vi "No GyroScope Acc Test.vi"() -> ()   [LabVIEW 2019]
uses:
  <vilib>/Platform/TimedLoop/XDataNode/timing_clust.ctl
  <vilib>/Platform/TimedLoop/XDataNode/nitl_modes.ctl
  <vilib>/Platform/TimedLoop/XDataNode/wakeup.ctl
  <vilib>/FPGAPlugInAG/cRIO-9065/niLvFpga_Open_cRIO-9065.vi
  <vilib>/rvi/interface/common/dynamic/niFpgaDynamicAddResources.vi
  <vilib>/Utility/error.llb/Error Cluster From Error Code.vi
  <vilib>/rvi/errors/niLvFpgaAdjustHostInterfaceError.vi
  <vilib>/FPGAPlugInAG/Dynamic/niLvFpga_Run_Dynamic.vi
  <vilib>/FPGAPlugInAG/Dynamic/niLvFpga_Abort_Dynamic.vi
  <vilib>/platform/TimedLoop/XDataNode/XDataNode.xnode
  <vilib>/rvi/interface/nirviOpenFPGA/nirviOpenFPGA.xnode
  FPGA Bitfiles/crio9065control_FPGATarget_3motionboardtest_jcOy0Y5QmHo.lvbitx
  <vilib>/rvi/interface/nirviReadWriteControl/nirviReadWriteControl.xnode
  <vilib>/rvi/interface/nirviMethod/nirviMethod.xnode
  NiFpgaLv.dll
  <vilib>/rvi/interface/Simulation/niFpgaSimulationCallBeginRW.vi
  <vilib>/Platform/TimedLoop/XDataNode/XDNodeRunTimeDep.lvlib
  <vilib>/Analysis/NI_AALPro.lvlib
panel:
  out "Axis 3 Real Acceleration Graph":cluster{i32[], "Ideal Acc":dbl[]}[](graph)
  out "Axis 2 Real Acceleration Graph":cluster{i32[], "Ideal Acc":dbl[]}[](graph)
  out "Axis 3 Real Velocity Graph":cluster{i32[], "Ideal Velocity":dbl[]}[](graph)
  out "Axis 2 Real Velocity Graph":cluster{i32[], "Ideal Velocity":dbl[]}[](graph)
  out "Axis 1 Real Acceleration Graph":cluster{i32[], "dX/dt":dbl[]}[](graph)
  out "Axis 1 Real Velocity Graph":cluster{i32[], "Ideal Velocity":dbl[]}[](graph)
  out "Axis 1":cluster{i32[], "Ideal Move":dbl[]}[](graph)
  out "Axis 3":cluster{i32[], "Ideal Move":dbl[]}[](graph)
  out "Axis 2":cluster{i32[], "Ideal Move":dbl[]}[](graph)
  in  "Period":i64=10
  in  "stop":bool
  out "time loop error":errorcluster
  out "Axis 1 速率 (1mm/s)":dbl
  out "Real Period":u32
  out "沖壓":bool
  out "結束了":bool
  out "Voltage\nOutput":dbl
  out "Voltage\nOutput 2":dbl
  out "Voltage\nOutput 3":dbl
  out "Axis 2 速率 (1mm/s)":dbl
  out "Axis 3 速率 (1mm/s)":dbl
  out "shutdown error":errorcluster
  in  "Tab Control":enum32{"Axis Control"}(tab)
  in  "Axis 1~3 Servo on?":bool
  out "Axis 3 Backward Limit":bool
  out "Axis 3 Backward Limit 2":bool
  out "Axis 2 Backward Limit":bool
  out "Axis 2 Backward Limit 2":bool
  in  "Axis 3 Alarm Reset":bool
  in  "Axis 2 Alarm Reset":bool
  in  "Axis 3 Position Reset":bool
  in  "Axis 2 Position Reset":bool
  in  "Axis 1 Alarm Reset":bool
  in  "Axis 1 Position Reset":bool
  in  "Axis 3 Speed":fxp<+/-,64,32>
  in  "Axis 2 Speed":fxp<+/-,64,32>
  out "Axis 3 Encoder Position (Counts)":i32
  out "Axis 2 Encoder Position (Counts)":i32
  out "Axis 1 Encoder Position (Counts)":i32
  in  "Axis 1 Spped":fxp<+/-,64,32>
  in  "Axis 2 Servo on?":bool
  in  "Axis 3 Servo on?":bool
  in  "Axis 1 Servo on?":bool
  out "Axis 1 Forward Limit":bool
  out "Axis 1 Backward Limit":bool
  out "Timed Out?":bool
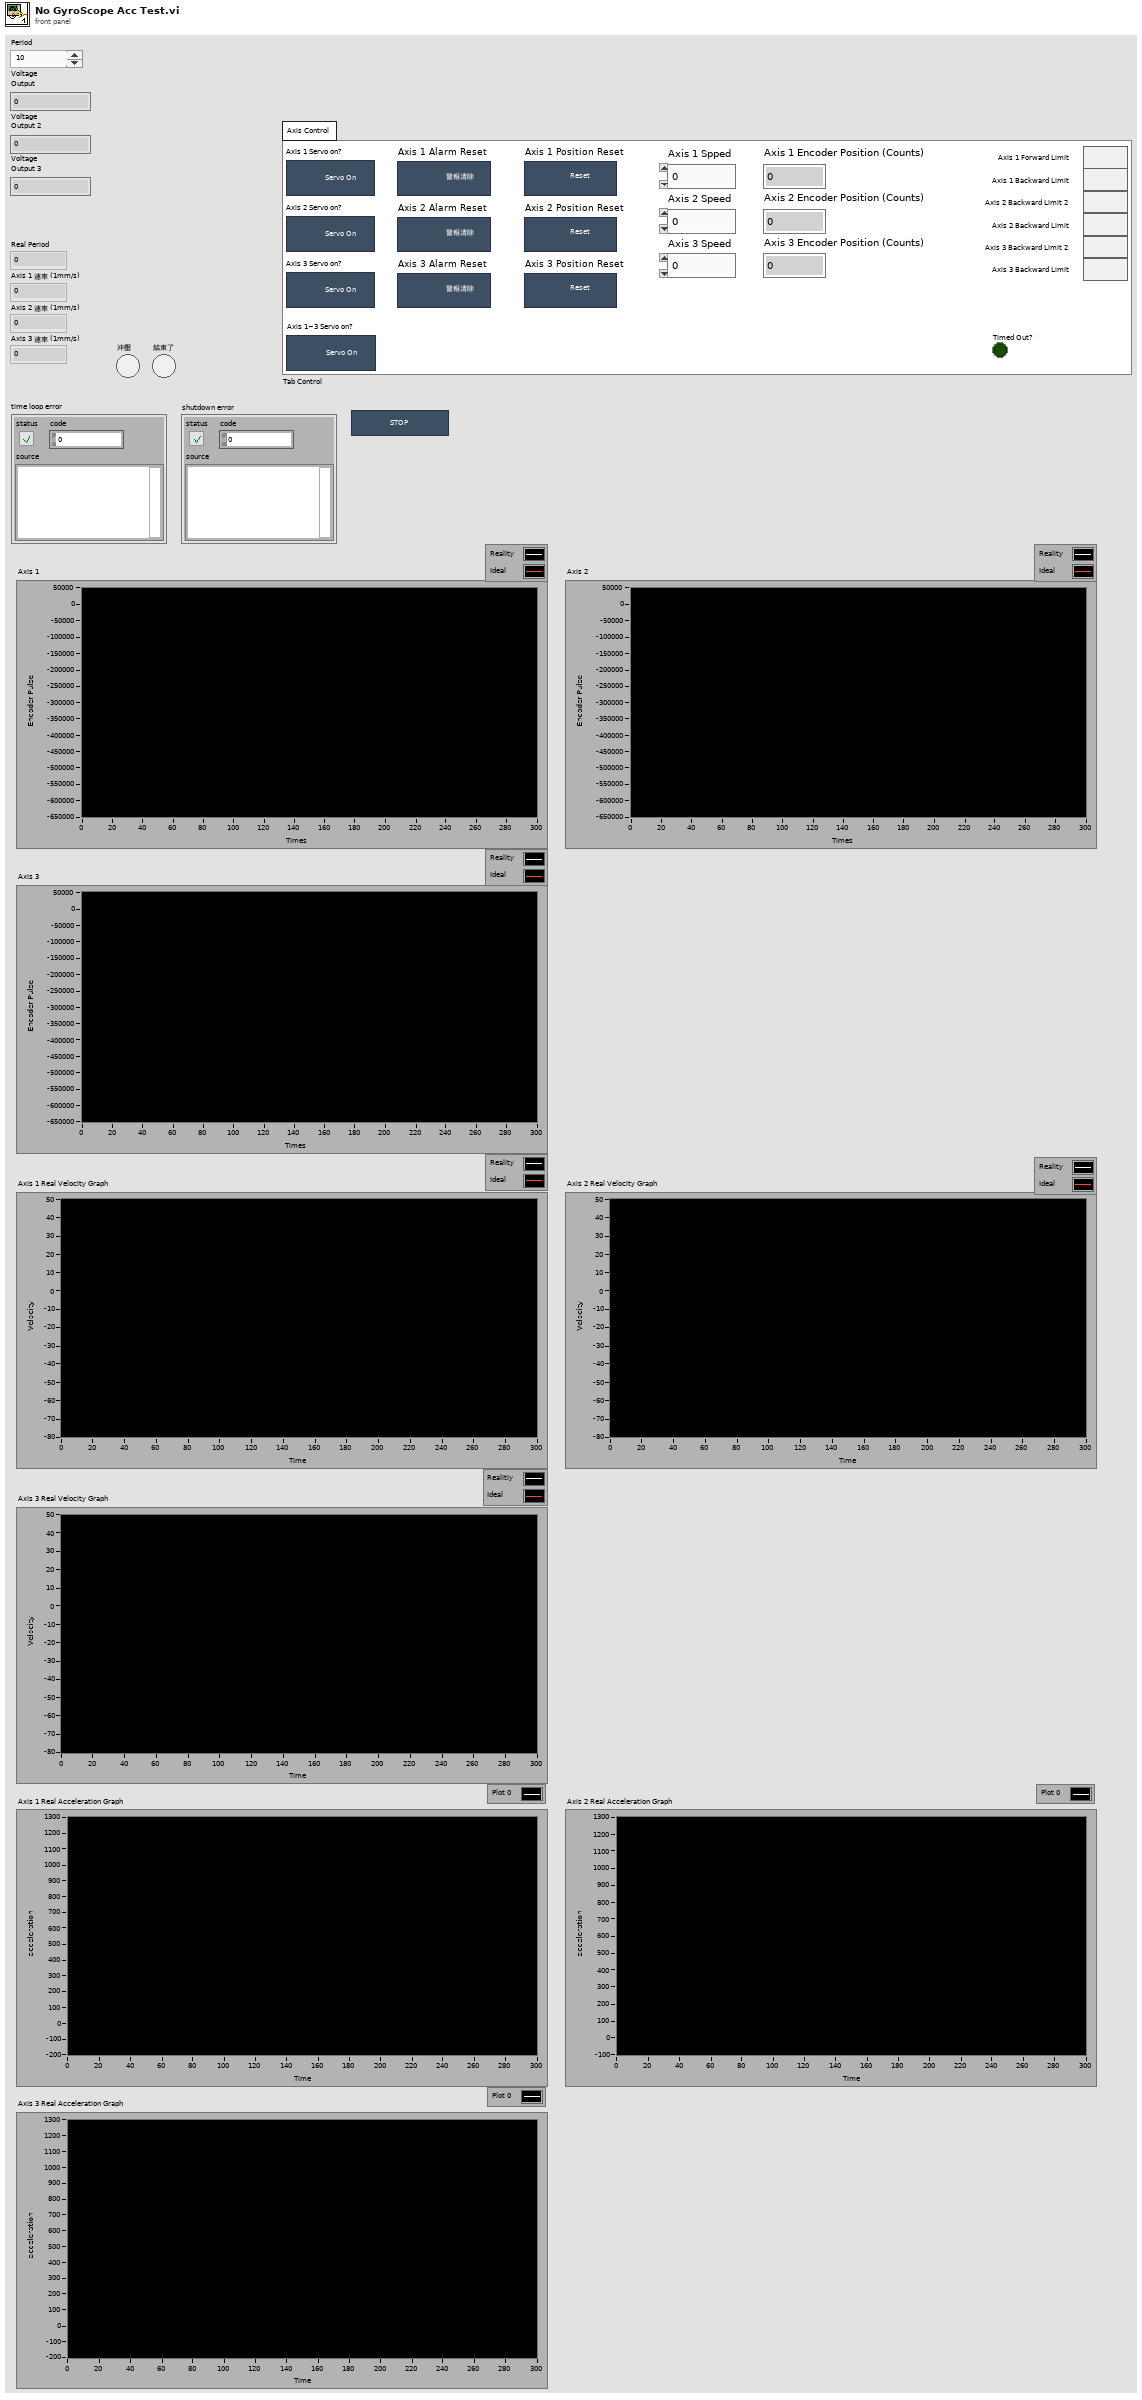
[diagram p1: front panel]
types:
  T1 = enum16{"open", "replace", "create", "open or create", "replace or create", "replace or create with confirmation"}
  T2 = cluster{"Acceleration 1":dbl, "Acceleration 2":dbl, "Acceleration 3":dbl, "Acceleration 4":dbl, "Acceleration 5":dbl, "Acceleration 6":dbl, "Acceleration 7":dbl, "Acceleration 8":dbl}
  T3 = cluster{"Time 1":dbl, "Time 2":dbl, "Time 3":dbl, "Time 4":dbl, "Time 5":dbl, "Time 6":dbl, "Time 7":dbl, "Time 8":dbl}
  T4 = typedef "XDNodeRunTimeDep.lvlib/timing_clust.ctl" = cluster{"Expected End [f-1]":u64, "Actual End [f-1]":u64, "Finished Late? [f-1]":bool, "Expected End [i-1]":u64, "Actual End [i-1]":u64, "Finished Late? [i-1]":bool, "Expected Start [i]":u64, "Actual Start [i]":u64, "Expected Start [f]":u64, "Actual Start [f]":u64, "Source Name":string, "Structure Name":string, "Period":i64, "Deadline":i64, "Offset":i64, "Start":i64, "Priority":i32, "Timeout":i32, "Mode":T5, "Wakeup Reason":T6, "Error":errorcluster, "Source Type":string, "Secondary Source Type":string, "Global End Time":u64, "Global Start Time":u64, "Frame Duration":u64, "Iteration Duration":u64, "Assigned CPU":i32, "I/O Scan Engine Mode":u32}
  T5 = typedef "XDNodeRunTimeDep.lvlib/nitl_modes.ctl" = enum32{"No Change", "Process missed periods, maintain original phase", "Discard missed periods, maintain original phase", "Process missed periods, ignore original phase", "Discard missed periods, ignore original phase"}
  T6 = typedef "XDNodeRunTimeDep.lvlib/wakeup.ctl" = enum32{"Normal", "Aborted", "Asynchronous wakeup", "Timing source error", "Timed loop error", "Timeout"}
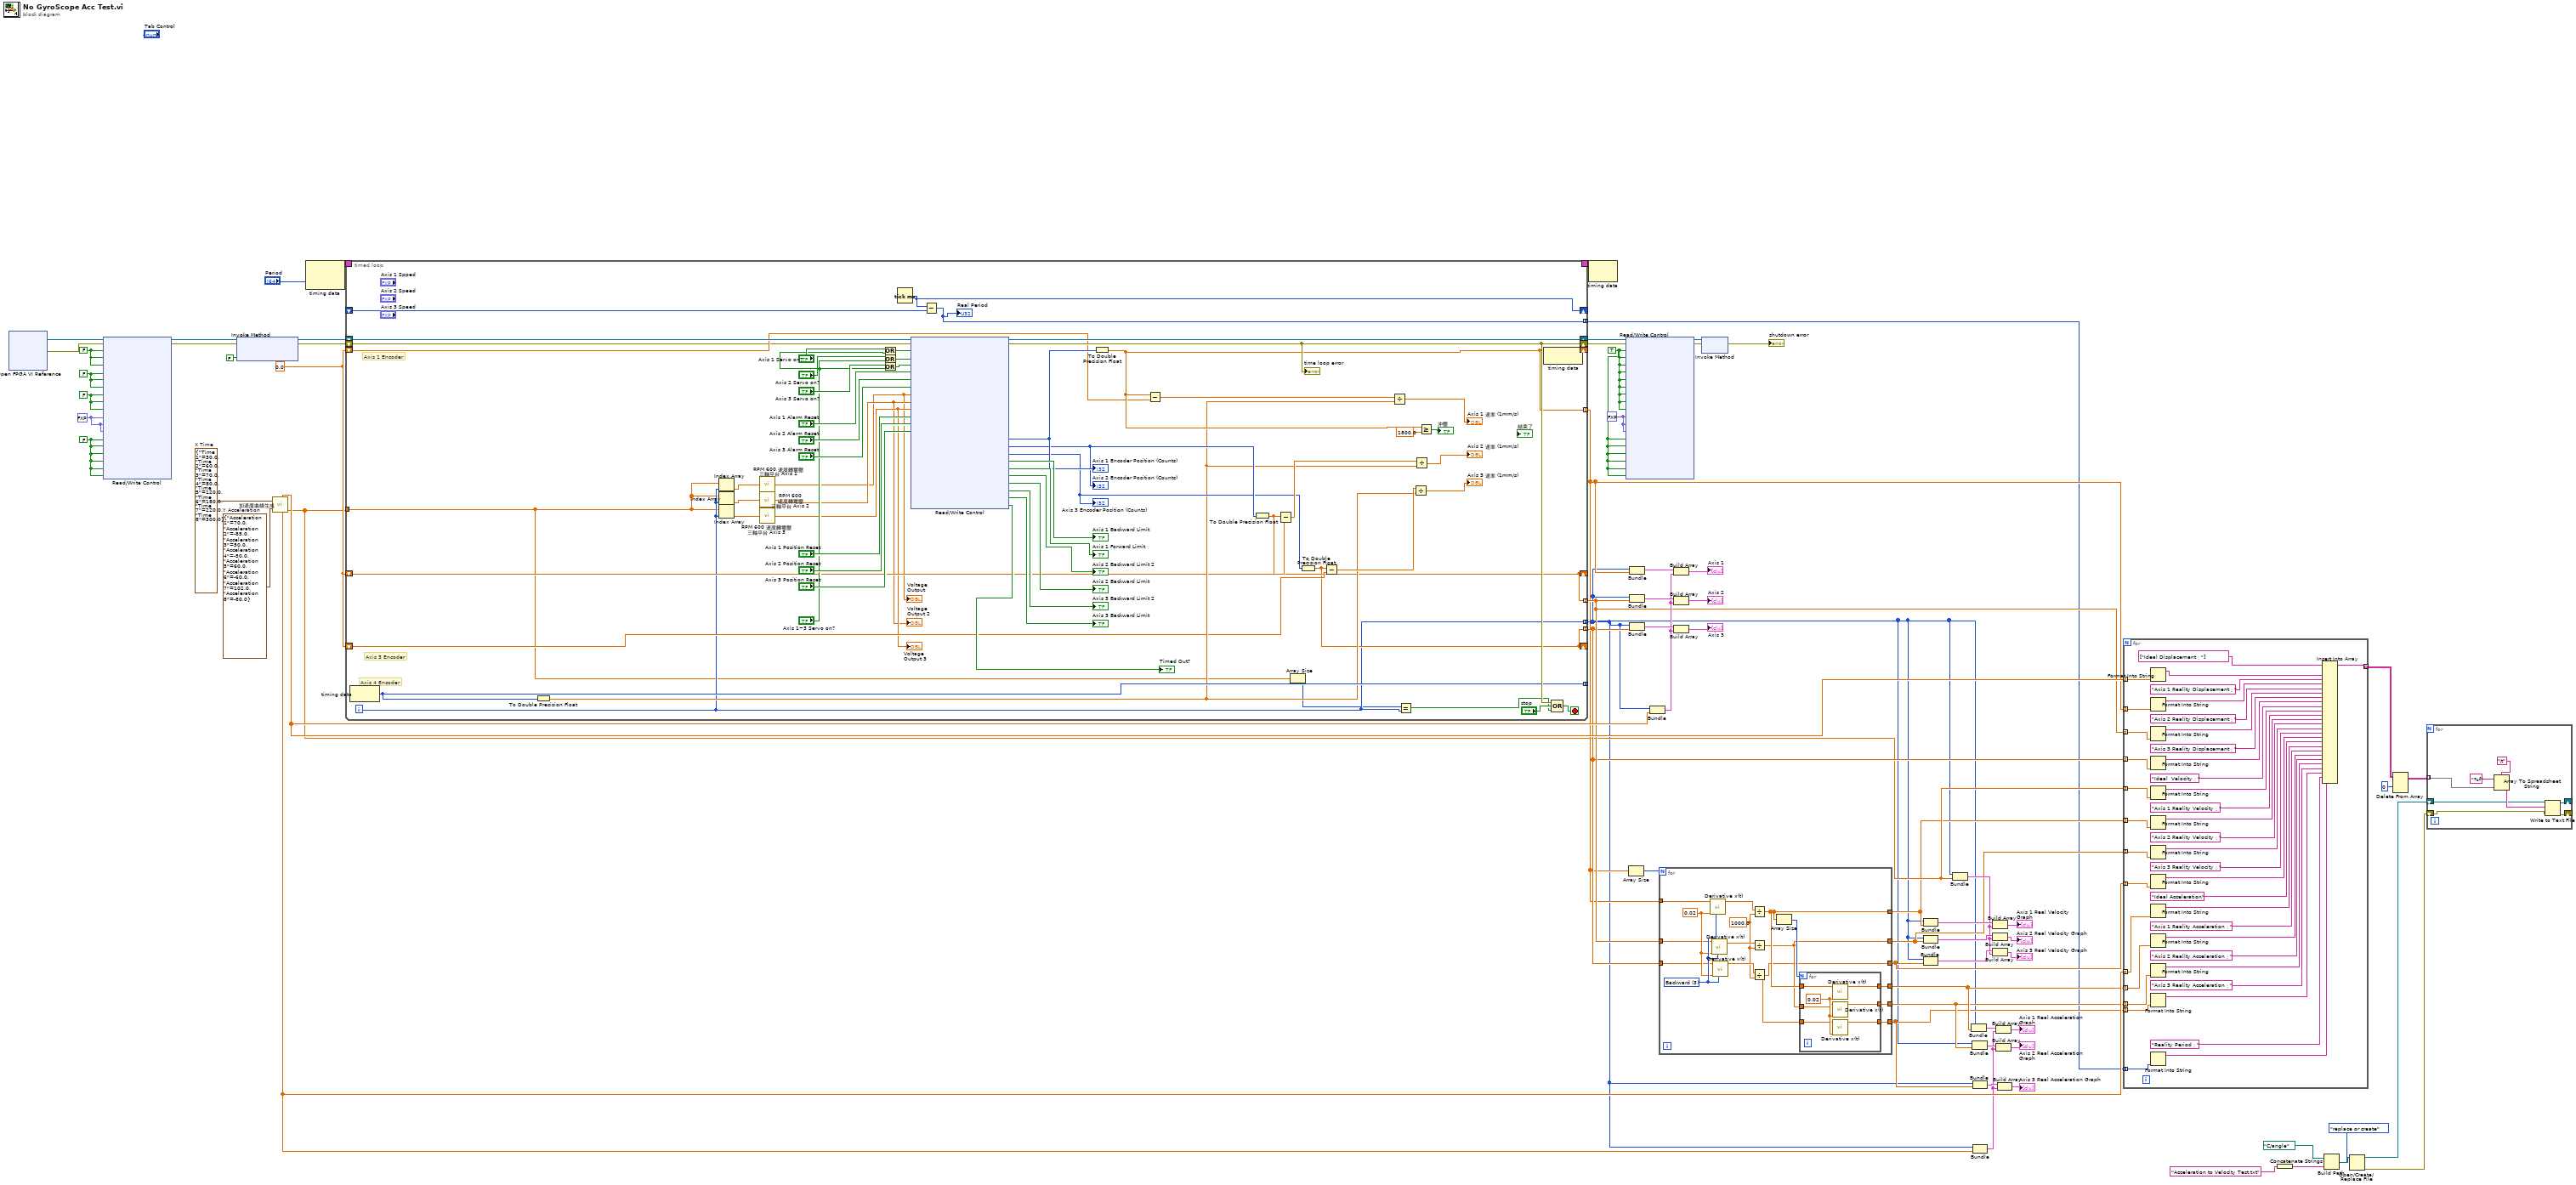
[diagram p0: block diagram]
diagram:
  w48 = T2 {"Acceleration 1"=70.0, "Acceleration 2"=-85.0, "Acceleration 3"=50.0, "Acceleration 4"=-50.0, "Acceleration 5"=60.0, "Acceleration 6"=-60.0, "Acceleration 7"=102.0, "Acceleration 8"=-80.0}  # Y Acceleration
  w50 = T3 {"Time 1"=30.0, "Time 2"=60.0, "Time 3"=70.0, "Time 4"=80.0, "Time 5"=120.0, "Time 6"=180.0, "Time 7"=220.0, "Time 8"=300.0}  # X Time
  w52 = FALSE
  w54 = FALSE
  w60 = 0.0
  w58 = fxp<+,1,1> 0.0
  w57 = TRUE
  w55 = FALSE
  w53 = fxp<+,1,1> 0.0
  w56 = FALSE
  n1 = xnode "Open FPGA VI Reference"() -> ("FPGA VI Reference Out"=w51:refnum<k20>, "error out"=w1:errorcluster)  [unwired: 2 in]
  n2 = xnode "Read/Write Control"("FPGA VI Reference In"=w51, "error in"=w1, "Axis 1 Servo on?"=w56, "Axis 2 Servo on?"=w56, "Axis 3 Servo on?"=w56, "Axis 1 Alarm Reset"=w55, "Axis 2 Alarm Reset"=w55, "Axis 3 Alarm Reset"=w55, "Axis 1 Position Reset"=w54, "Axis 2 Position Reset"=w54, "Axis 3 Position Reset"=w54, "Axis 1 Voltage In"=w53, "Axis 2 Voltage In"=w53, "Axis 3 Voltage In"=w53, "Axis 1 Backward Limit"=w52, "Axis 1 Forward Limit"=w52, "Axis 2 Forward Limit"=w52, "Axis 2 Backward Limit"=w52, "Axis 3 ForWard Limit"=w52, "Axis 3 Backward Limit"=w52) -> ("FPGA VI Reference Out"=w69:refnum<k20>, "error out"=w68:errorcluster)
  n3 = xnode "Invoke Method"("FPGA VI Reference In"=w69, "error in"=w68, "Wait Until Done (F)"=FALSE) -> ("FPGA VI Reference Out"=w66:refnum<k20>, "error out"=w2:errorcluster)
  n4 = call "加速度曲線生成.vi"("X Time"=w50, "Y Velocity"=w48) -> ("Ideal Move"=w26:dbl[], "Ideal Acc"=w9:dbl[], "Ideal Velocity"=w22:dbl[])  [unwired: 3 out]
  n5 = node-c288("Period") -> (w71:T4)  [unwired: 1 in]
  n6 = timed-loop {
    shift-right: [w128] -> w62
    shift-left: w66 -> [w127]
    shift-right: [w95] -> w63
    shift-left: w2 -> [w72]
    timing: w71 -> [_]
    timing-out: [_] -> w70
    shift-right: [w90] -> _
    shift-left: w60 -> [w89]
    tunnel: [w94] -> _ mode=indexing
    shift-right: [w124] -> _
    shift-left: _ -> [w125]
    tunnel: [w84] -> w5 mode=indexing
    shift-right: [w83] -> _
    shift-left: w60 -> [w86]
    shift-right: [w82] -> _
    shift-left: w60 -> [w87]
    tunnel: [w81] -> w3 mode=indexing
    tunnel: [w90] -> w23 mode=indexing
    tunnel: [w83] -> w25 mode=indexing
    tunnel: [w82] -> w24 mode=indexing
    tunnel: w22 -> [w73]
    i -> [w81]
    stop <- w126 stop-if-true
    # "Axis 3 Encoder"
    # "Axis 4 Encoder"
    # "Axis 1 Encoder"
    n7 = node-c288() -> (w94:i64)  [unwired: 1 in]
    n8 = To Double Precision Float(number=w94) -> (double precision float=w88:dbl)
    n9 = Index Array(array=w73, index=w81) -> (element=w78:dbl)
    n10 = Index Array(array=w73, index=w81) -> (element=w77:dbl)
    n11 = Index Array(array=w73, index=w81) -> (element=w79:dbl)
    n12 = call "RPM 600 速度轉電壓 三軸平台 Axis 1.vi"("Speed (1mm/s)"=w78) -> ("Voltage\nOutput"=w74:dbl)
    "Voltage\nOutput" <- w74
    n13 = call "RPM 600 速度轉電壓 三軸平台 Axis 2.vi"("Speed (1mm/s)"=w77) -> ("Voltage\nOutput"=w75:dbl)
    "Voltage\nOutput 2" <- w75
    n14 = call "RPM 600 速度轉電壓 三軸平台 Axis 3.vi"("Speed (1mm/s)"=w79) -> ("Voltage\nOutput"=w76:dbl)
    "Voltage\nOutput 3" <- w76
    n15 = Or(x="Axis 1 Servo on?", y="Axis 1~3 Servo on?") -> (x .or. y?=w107:bool)
    n16 = Or(x="Axis 2 Servo on?", y="Axis 1~3 Servo on?") -> (x .or. y?=w104:bool)
    n17 = Or(x="Axis 3 Servo on?", y="Axis 1~3 Servo on?") -> (x .or. y?=w102:bool)
    n18 = Tick Count (ms)() -> (millisecond timer value=w124:u32)
    n19 = xnode "Read/Write Control"("FPGA VI Reference In"=w127, "error in"=w72, "Axis 1 Servo on?"=w107, "Axis 2 Servo on?"=w104, "Axis 3 Servo on?"=w102, "Axis 1 Alarm Reset"="Axis 1 Alarm Reset", "Axis 2 Alarm Reset"="Axis 2 Alarm Reset", "Axis 3 Alarm Reset"="Axis 3 Alarm Reset", "Axis 1 Voltage In"=w74, "Axis 2 Voltage In"=w75, "Axis 3 Voltage In"=w76, "Axis 1 Position Reset"="Axis 1 Position Reset", "Axis 2 Position Reset"="Axis 2 Position Reset", "Axis 3 Position Reset"="Axis 3 Position Reset") -> ("FPGA VI Reference Out"=w128:refnum<k20>, "error out"=w95:errorcluster, "Axis 1 Encoder Position (Counts)"=w100:i32, "Axis 2 Encoder Position (Counts)"=w98:i32, "Axis 3 Encoder Position (Counts)"=w97:i32, "Axis 1 Backward Limit"=→"Axis 1 Backward Limit":bool, "Axis 1 Forward Limit"=→"Axis 1 Forward Limit":bool, "Axis 2 Backward Limit"=→"Axis 2 Backward Limit 2":bool, "Axis 2 Forward Limit"=→"Axis 2 Backward Limit":bool, "Axis 3 Backward Limit"=→"Axis 3 Backward Limit 2":bool, "Axis 3 ForWard Limit"=→"Axis 3 Backward Limit":bool, "Timed Out?"=→"Timed Out?":bool)
    "time loop error" <- w95
    "Axis 1 Encoder Position (Counts)" <- w100
    "Axis 2 Encoder Position (Counts)" <- w98
    "Axis 3 Encoder Position (Counts)" <- w97
    n20 = Subtract(x=w124, y=w125) -> (x-y=w84:u32)
    "Real Period" <- w84
    n21 = To Double Precision Float(number=w100) -> (double precision float=w90:dbl)
    n22 = Subtract(x=w90, y=w89) -> (x-y=w129:dbl)
    n23 = To Double Precision Float(number=w98) -> (double precision float=w83:dbl)
    n24 = Subtract(x=w83, y=w86) -> (x-y=w99:dbl)
    n25 = Array Size(array=w73) -> (size(s)=w80:i32)
    n26 = To Double Precision Float(number=w97) -> (double precision float=w82:dbl)
    n27 = Subtract(x=w82, y=w87) -> (x-y=w96:dbl)
    n28 = Divide(x=w129, y=w88) -> (x/y=→"Axis 1 速率 (1mm/s)":dbl)
    n29 = Equal?(x=w80, y=w81) -> (x = y?=w85:bool)
    n30 = Divide(x=w96, y=w88) -> (x/y=→"Axis 3 速率 (1mm/s)":dbl)
    n31 = Divide(x=w99, y=w88) -> (x/y=→"Axis 2 速率 (1mm/s)":dbl)
    n32 = Greater Or Equal?(x=w90, y=1800.0) -> (x >= y?=→"沖壓":bool)
    n33 = node-c288() -> ()  [unwired: 1 in, 1 out]
    n34 = Compound Arithmetic op=OR(w95, "stop", w85) -> (w126:bool)
  }
  n35 = node-c288(w70) -> ()  [unwired: 1 out]
  n36 = xnode "Read/Write Control"("FPGA VI Reference In"=w62, "error in"=w63, "Axis 1 Servo on?"=w57, "Axis 2 Servo on?"=w57, "Axis 3 Servo on?"=w57, "Axis 1 Alarm Reset"=w57, "Axis 2 Alarm Reset"=w57, "Axis 3 Alarm Reset"=w57, "Axis 1 Position Reset"=w57, "Axis 2 Position Reset"=w57, "Axis 3 Position Reset"=w57, "Axis 1 Voltage In"=w58, "Axis 2 Voltage In"=w58, "Axis 3 Voltage In"=w58, "Axis 1 Backward Limit"=w57, "Axis 1 Forward Limit"=w57, "Axis 2 Forward Limit"=w57, "Axis 2 Backward Limit"=w57, "Axis 3 ForWard Limit"=w57, "Axis 3 Backward Limit"=w57) -> ("FPGA VI Reference Out"=w65:refnum<k20>, "error out"=w64:errorcluster)
  n37 = Array Size(array=w23) -> (size(s)=w49:i32)
  n38 = Bundle(w3, w23) -> (w40:cluster{i32[], dbl[]})  [unwired: 1 in]
  n39 = Bundle(w3, w25) -> (w39:cluster{i32[], dbl[]})  [unwired: 1 in]
  n40 = Bundle(w3, w24) -> (w38:cluster{i32[], dbl[]})  [unwired: 1 in]
  n41 = Bundle(w3, "Ideal Move"=w26) -> (w37:cluster{i32[], "Ideal Move":dbl[]})  [unwired: 1 in]
  n42 = for {
    N: w49 -> [_]
    tunnel: w23 -> [w148]
    tunnel: [w146] -> w21
    tunnel: [w144] -> w8
    tunnel: w25 -> [w141]
    tunnel: w24 -> [w140]
    tunnel: [w139] -> w7
    tunnel: [w138] -> w6
    tunnel: [w134] -> w20
    tunnel: [w133] -> w19
    w143 = u16 3 items=["2nd Order Central", "4th Order Central", "Forward", "Backward"] ("method")
    w135 = 1000.0 ("dt")
    w142 = 0.02 ("dt")
    n43 = call <vilib>:"Derivative x(t).vi"("method"=w143, "dt"=w142, "X"=w148) -> ("dX/dt"=w147:dbl[])  [unwired: 7 in, 1 out]
    n44 = call <vilib>:"Derivative x(t).vi"("method"=w143, "dt"=w142, "X"=w141) -> ("dX/dt"=w137:dbl[])  [unwired: 7 in, 1 out]
    n45 = call <vilib>:"Derivative x(t).vi"("method"=w143, "dt"=w142, "X"=w140) -> ("dX/dt"=w136:dbl[])  [unwired: 7 in, 1 out]
    n46 = Divide(x=w147, y=w135) -> (x/y=w146:dbl[])
    n47 = Divide(x=w137, y=w135) -> (x/y=w134:dbl[])
    n48 = Divide(x=w136, y=w135) -> (x/y=w133:dbl[])
    n49 = Array Size(array=w146) -> (size(s)=w145:i32)
    n50 = for {
      N: w145 -> [_]
      tunnel: w146 -> [w154]
      tunnel: [w155] -> w144
      tunnel: w134 -> [w152]
      tunnel: w133 -> [w151]
      tunnel: [w150] -> w139
      tunnel: [w149] -> w138
      w153 = 0.02 ("dt")
      n51 = call <vilib>:"Derivative x(t).vi"("dt"=w153, "X"=w154) -> ("dX/dt"=w155:dbl[])  [unwired: 8 in, 1 out]
      n52 = call <vilib>:"Derivative x(t).vi"("dt"=w153, "X"=w152) -> ("dX/dt"=w150:dbl[])  [unwired: 8 in, 1 out]
      n53 = call <vilib>:"Derivative x(t).vi"("dt"=w153, "X"=w151) -> ("dX/dt"=w149:dbl[])  [unwired: 8 in, 1 out]
    }
  }
  n54 = Build Array(w40, w37) -> (→"Axis 1":cluster{i32[], "Ideal Move":dbl[]}[])
  n55 = Build Array(w39, w37) -> (→"Axis 2":cluster{i32[], "Ideal Move":dbl[]}[])
  n56 = Build Array(w38, w37) -> (→"Axis 3":cluster{i32[], "Ideal Move":dbl[]}[])
  n57 = xnode "Invoke Method"("FPGA VI Reference In"=w65, "error in"=w64) -> ("error out"=→"shutdown error":errorcluster)  [unwired: 1 out]
  n58 = Bundle(w3, w21) -> (w47:cluster{i32[], dbl[]})  [unwired: 1 in]
  n59 = Bundle(w3, w20) -> (w46:cluster{i32[], dbl[]})  [unwired: 1 in]
  n60 = Bundle(w3, w19) -> (w45:cluster{i32[], dbl[]})  [unwired: 1 in]
  n61 = Bundle(w3, "Ideal Velocity"=w22) -> (w41:cluster{i32[], "Ideal Velocity":dbl[]})  [unwired: 1 in]
  n62 = Bundle(w3, "dX/dt"=w8) -> (w14:cluster{i32[], "dX/dt":dbl[]})  [unwired: 1 in]
  n63 = Bundle(w3, "dX/dt"=w7) -> (w13:cluster{i32[], "dX/dt":dbl[]})  [unwired: 1 in]
  n64 = Bundle(w3, "dX/dt"=w6) -> (w12:cluster{i32[], "dX/dt":dbl[]})  [unwired: 1 in]
  n65 = Bundle(w3, "Ideal Acc"=w9) -> (w4:cluster{i32[], "Ideal Acc":dbl[]})  [unwired: 1 in]
  n66 = Build Array(w47, w41) -> (→"Axis 1 Real Velocity Graph":cluster{i32[], "Ideal Velocity":dbl[]}[])
  n67 = Build Array(w46, w41) -> (→"Axis 2 Real Velocity Graph":cluster{i32[], "Ideal Velocity":dbl[]}[])
  n68 = Build Array(w45, w41) -> (→"Axis 3 Real Velocity Graph":cluster{i32[], "Ideal Velocity":dbl[]}[])
  n69 = Build Array(w14, w4) -> (→"Axis 1 Real Acceleration Graph":cluster{i32[], "Ideal Acc":dbl[]}[])
  n70 = Build Array(w13, w4) -> (→"Axis 2 Real Acceleration Graph":cluster{i32[], "Ideal Acc":dbl[]}[])
  n71 = Build Array(w12, w4) -> (→"Axis 3 Real Acceleration Graph":cluster{i32[], "Ideal Acc":dbl[]}[])
  n72 = for {
    tunnel: [w194] -> w18 mode=indexing
    tunnel: w26 -> [w191] mode=indexing
    tunnel: w23 -> [w190] mode=indexing
    tunnel: w25 -> [w176] mode=indexing
    tunnel: w24 -> [w175] mode=indexing
    tunnel: w22 -> [w174] mode=indexing
    tunnel: w21 -> [w173] mode=indexing
    tunnel: w20 -> [w172] mode=indexing
    tunnel: w19 -> [w171] mode=indexing
    tunnel: w9 -> [w170] mode=indexing
    tunnel: w8 -> [w161] mode=indexing
    tunnel: w7 -> [w160] mode=indexing
    tunnel: w6 -> [w159] mode=indexing
    tunnel: w5 -> [w158] mode=indexing
    n73 = Format Into String(w191) -> (resulting string=w193:string)  [unwired: 3 in, 1 out]
    n74 = Format Into String(w190) -> (resulting string=w189:string)  [unwired: 3 in, 1 out]
    n75 = Format Into String(w176) -> (resulting string=w187:string)  [unwired: 3 in, 1 out]
    n76 = Format Into String(w175) -> (resulting string=w185:string)  [unwired: 3 in, 1 out]
    n77 = Format Into String(w174) -> (resulting string=w183:string)  [unwired: 3 in, 1 out]
    n78 = Format Into String(w173) -> (resulting string=w181:string)  [unwired: 3 in, 1 out]
    n79 = Format Into String(w172) -> (resulting string=w179:string)  [unwired: 3 in, 1 out]
    n80 = Format Into String(w171) -> (resulting string=w177:string)  [unwired: 3 in, 1 out]
    n81 = Format Into String(w170) -> (resulting string=w168:string)  [unwired: 3 in, 1 out]
    n82 = Format Into String(w161) -> (resulting string=w166:string)  [unwired: 3 in, 1 out]
    n83 = Format Into String(w160) -> (resulting string=w164:string)  [unwired: 3 in, 1 out]
    n84 = Format Into String(w159) -> (resulting string=w162:string)  [unwired: 3 in, 1 out]
    n85 = Format Into String(w158) -> (resulting string=w156:string)  [unwired: 3 in, 1 out]
    n86 = Insert Into Array(array=string[] ["Ideal Displacement："], new element #1=w193, new element #2="Axis 1 Reality Displacement：", new element #3=w189, new element #4="Axis 2 Reality Displacement：", new element #5=w187, new element #6="Axis 3 Reality Displacement：", new element #7=w185, new element #8="Ideal  Velocity：", new element #9=w183, new element #10="Axis 1 Reality Velocity：", new element #11=w181, new element #12="Axis 2 Reality Velocity：", new element #13=w179, new element #14="Axis 3 Reality Velocity：", new element #15=w177, new element #16="Ideal Acceleration", new element #17=w168, new element #18="Axis 1 Reality Acceleration：", new element #19=w166, new element #20="Axis 2 Reality Acceleration：", new element #21=w164, new element #22="Axis 3 Reality Acceleration：", new element #23=w162, new element #24="Reality Period：", new element #25=w156) -> (w194:string[])  [unwired: 1 in]
  }
  n87 = Concatenate Strings("Acceleration to Velocity Test.txt" ("element")) -> (w32:string)
  n88 = Build Path(base path=path "C:/angle", name or relative path=w32) -> (appended path=w33:path)
  n89 = Open/Create/Replace File(file path (use dialog)=w33, operation (0:open)=T1."replace or create") -> (refnum out=w17:refnum<file>, error out=w16:errorcluster)  [unwired: 4 in, 1 out]
  n90 = Delete From Array(array=w18, index (row)=0) -> (array with subset deleted=w28:string[][])  [unwired: 2 in, 1 out]
  n91 = for {
    shift-right: [w197] -> _
    shift-left: w17 -> [w200]
    shift-right: [w198] -> _
    shift-left: w16 -> [w199]
    tunnel: w28 -> [w196] mode=indexing
    n92 = Array To Spreadsheet String(delimiter (Tab)="\t", array=w196, 3:"%f" ("format string")) -> (spreadsheet string=w201:string)
    n93 = Write to Text File(file (use dialog)=w200, text=w201, error in=w199) -> (refnum out=w197:refnum<file>, error out=w198:errorcluster)  [unwired: 1 in, 1 out]
  }
